vi "Build No-Reply Asynchronous Message with Arguments.vi"(5 "State With Arguments":string, 7 "Arguments (\"\")":string, 9 "Target Module (\"\")":string) -> (6 "CSM Message String":string)   [LabVIEW 2017, in "Communicable State Machine.lvlib"]
doc: "Concatenates and generates CSM asynchronous message strings without reply. The message type symbol is `->|`, for example:\n\n Message >> Arguments ->| Target\n\n\n> [!NOTE] <b>Message Building API</b>\n>\n> This type of API is only used to concatenate message strings and does not send messages directly. The strings need to be merged into the CSM state queue, and the messages will be sent and the operation executed within the Parse State Queue++ VI. If you are familiar with CSM rules, you do not need to use this type of API. You can type the corresponding message string or operation string directly into the string.\n\n\n> [!NOTE] <b>Asynchronous Message</b>\n>\n> An asynchronous message is a type of message. After a CSM sends an asynchronous message, it immediately continues to execute subsequent code without waiting for the callee to complete message processing. Asynchronous messages are divided into Asynchronous Call (`->`) and Asynchronous Call without Reply (`->|`). The only difference is that with an Asynchronous Call without Reply (`->|`), the callee will not return the result to the caller after completing the operation.\n>\n> <b>Errors occurring at the Caller</b>:\n> - If the input target module is `\"\"`, a `NO Target Error` is generated.\n> - If the input module does not exist, a `Target Error` is generated.\n>\n> <b>Caller does not wait for return</b>:\n> - If the caller is a CSM module, it enters the `Async Message Posted` state after sending the message in the Parse State Queue++ VI.\n> - If it is an API call, it continues to execute subsequent code. The API can only send Asynchronous without Reply messages.\n>\n> <b>Return</b>:\n> - <b>If the caller is a CSM module</b>:\n> - Normally, it enters the `Async Response` state to handle the return. If an error occurs at the callee, this information is still the result of the message. It is handled in the `Async Response` state, and this error information can be obtained from Additional Information.\n> - If an error occurs at the caller, it causes the CSM state machine to enter the `Error Handler` module to handle the error.\n> - There is no return if the API can only send Asynchronous without Reply messages.\n\n\n> [!NOTE] <b>CSM Message Target Module Description</b>\n>\n> In Normal Mode, the target module for a CSM message is the specified module name.\n> System-level modules start with a `.` in their name. The target module for a CSM message includes the `.` in the name. For example, if the requested module name is `.System`, the target module for the CSM message is `.System`.\n> In Worker Mode, the target module for a CSM message can only be the overall module name, not the node name. For example, if the requested module name is `Worker#`, the target module for the CSM message is `Worker`.\n> In Chain of Responsibility Mode, the target module for a CSM message can only be the overall module name, not the node name. For example, if the requested module name is `Chain$1`, the target module for the CSM message is `Chain`.\n> In Chain of Responsibility Mode, a message is routed directly based on handling capability and priority (smaller number = higher priority) and is not passed sequentially across nodes.\n\n\n-- <b>Controls</b> --\n- <b>State with Arguments</b>: CSM state string.\n- <b>Arguments (\"\")</b>: Argument information. Arguments contained in <b>State with Arguments</b> will be replaced.\n- <b>Target Module (\"\")</b>: Target module. If empty, the default module in <b>State with Arguments</b> will be used.\n\n-- <b>Indicators</b> --\n- <b>CSM Message String</b>: Concatenated CSM message string."
uses:
  Communicable State Machine.lvlib
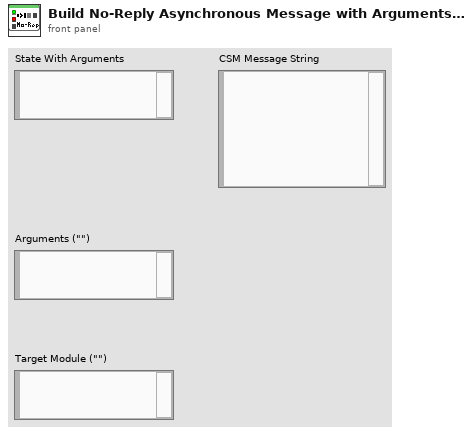
[diagram p1: front panel]
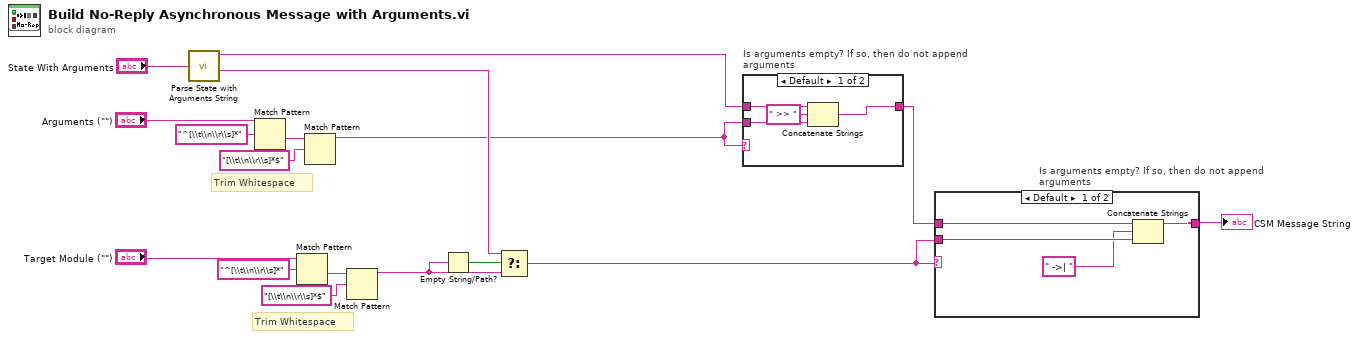
[diagram p0: block diagram]
diagram:
  # "Trim Whitespace"
  # "Trim Whitespace"
  n1 = call "Parse State with Arguments String.vi"("State With Arguments"="State With Arguments") -> ("State"=w3:string, "Target Module"=w8:string)  [unwired: 6 in, 2 out]
  n2 = Match Pattern(string="Arguments (\"\")", regular expression="^[\\t\\n\\r\\s]*") -> (after substring=w14:string)  [unwired: 1 in, 3 out]
  n3 = Match Pattern(string="Target Module (\"\")", regular expression="^[\\t\\n\\r\\s]*") -> (after substring=w11:string)  [unwired: 1 in, 3 out]
  n4 = Match Pattern(string=w14, regular expression="[\\t\\n\\r\\s]*$") -> (before substring=w1:string)  [unwired: 1 in, 3 out]
  n5 = Match Pattern(string=w11, regular expression="[\\t\\n\\r\\s]*$") -> (before substring=w7:string)  [unwired: 1 in, 3 out]
  n6 = Empty String/Path?(string/path=w7) -> (empty?=w9:bool)
  n7 = Select(t=w8, s=w9, f=w7) -> (s? t:f=w2:string)
  n8 = case "Is arguments empty? If so, then do not append arguments" shown="Default" w1 {
    tunnel: [w18 w22] -> w16
    tunnel: w3 -> [w21 w22]
    tunnel: w1 -> [w19 _]
    frame Default {
      n9 = Concatenate Strings(w21, " >> " ("string"), w19) -> (w18:string)
    }
    frame "" {
    }
  }
  n10 = case "Is arguments empty? If so, then do not append arguments" shown="Default" w2 {
    tunnel: [w24 w27] -> w17
    tunnel: w16 -> [w26 w27]
    tunnel: w2 -> [w25 _]
    frame Default {
      n11 = Concatenate Strings(w26, " ->| " ("string"), w25) -> (w24:string)
    }
    frame "" {
    }
  }
  "CSM Message String" <- w17
